vi "Is Concrete Class.vi"(0 "Vector 26GHz Path Group in":refnum<class "Vector 26GHz Path Group.lvclass">, 11 "error in (no error)":errorcluster) -> (4 "Vector 26GHz Path Group out":refnum<class "Vector 26GHz Path Group.lvclass">, 6 "Is Concrete Class?":bool, 15 "error out":errorcluster)   [LabVIEW 2023, in "RFFixtureCharact.RMM.lvlib" / "Vector 26GHz Path Group.lvclass"]
uses:
  Vector 26GHz Path Group.lvclass
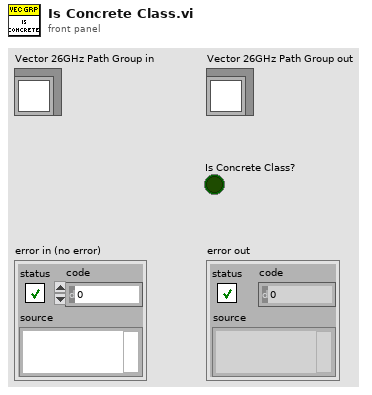
[diagram p1: front panel]
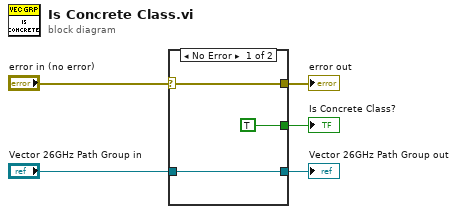
[diagram p0: block diagram]
diagram:
  n1 = case shown="No Error" "error in (no error)" {
    selector: "error in (no error)" -> [w7 w10]
    tunnel: [TRUE ("Is Concrete Class?") _] -> w3
    tunnel: [w7 w10] -> w1
    tunnel: [w6 w9] -> w4
    tunnel: "Vector 26GHz Path Group in" -> [w6 w9]
    frame No Error {
    }
    frame Error {
    }
  }
  "error out" <- w1
  "Vector 26GHz Path Group out" <- w4
  "Is Concrete Class?" <- w3
